vi "Start Up Procedure.vi"() -> ()   [LabVIEW 2015]
uses:
  <vilib>/DAQmx/write.llb/DAQmx Write (Digital Bool 1Line 1Point).vi
  <vilib>/DAQmx/miscellaneous.llb/DAQmx Fill In Error Info.vi
panel:
  out "PSU End of Charge":bool
  out "Start Button Pressed?":bool
  out "Earthed":bool
  out "System Reset pressed?":bool
  out "Safety System Interlock":bool
  out "HV On Relay":bool
  in  "Unlock Encloure Door":bool
  out "Enclosure Door Shut?":bool
  out "HV Enclosure OK":bool
  in  "Test HV Enclosure":bool
  out "Red Rack Enclosure OK":bool
  in  "Test Red Rack Enclosure":bool
  out "Emergency Stop OK":bool
  in  "Test Emergency Stop":bool
  out "Dump Switch Readback OK":bool
  in  "Test Dump Switch":bool
  in  "stop":bool
  out "LEDs OK":bool
  in  "Test LEDs":bool
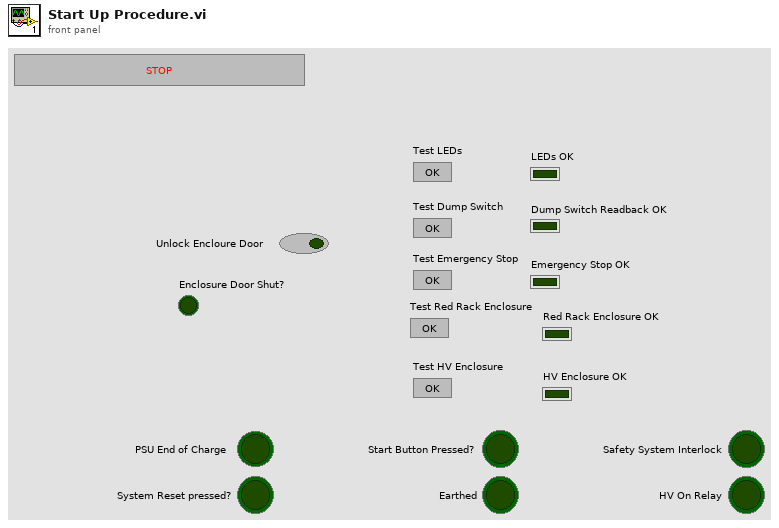
[diagram p1: front panel]
types:
  T1 = typedef "Semaphore RefNum" = refnum<k1>
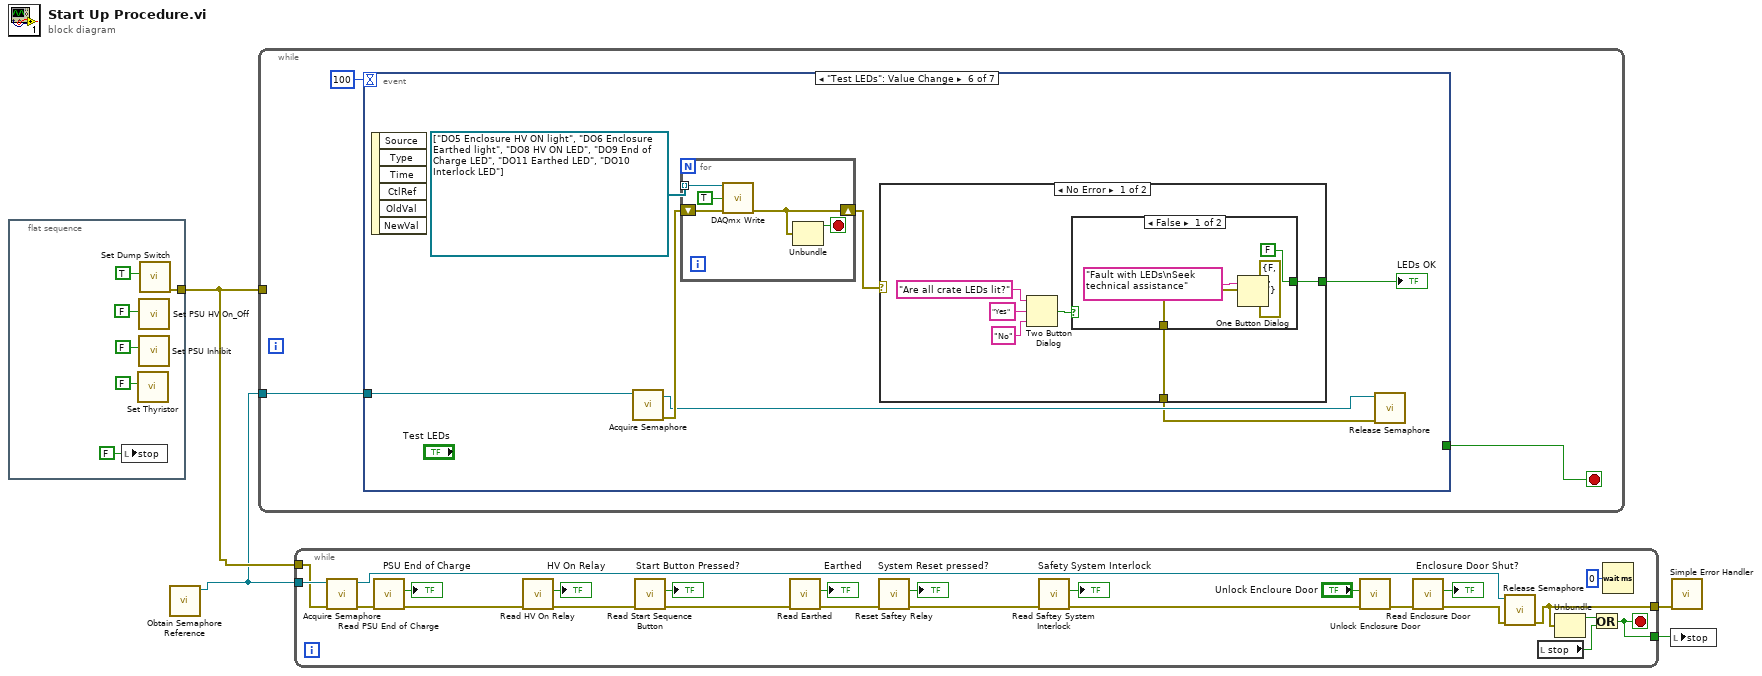
[diagram p0: block diagram]
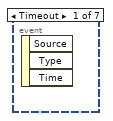
[diagram p2: hidden frame]
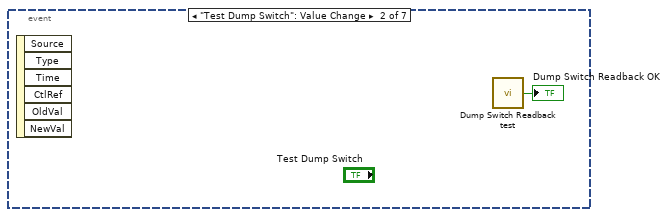
[diagram p3: hidden frame]
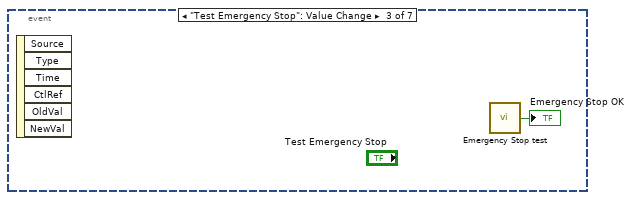
[diagram p4: hidden frame]
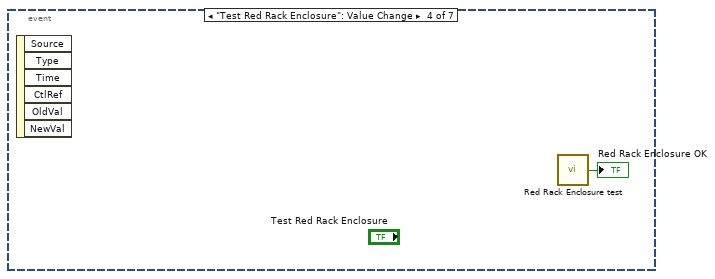
[diagram p5: hidden frame]
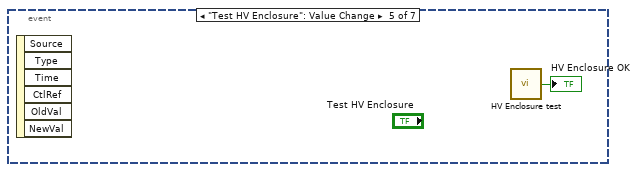
[diagram p6: hidden frame]
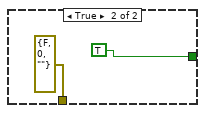
[diagram p7: hidden frame]
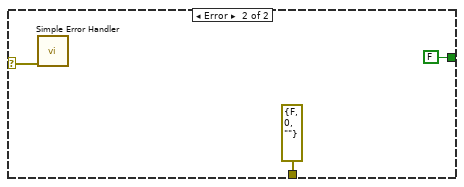
[diagram p8: hidden frame]
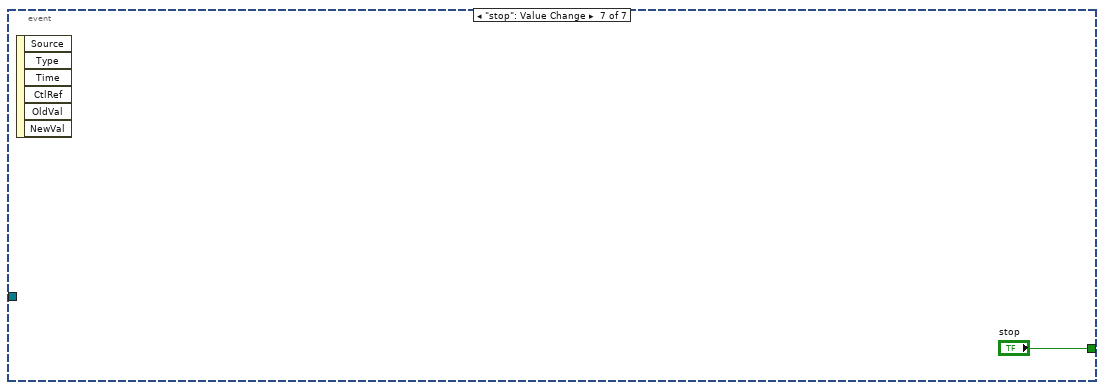
[diagram p9: hidden frame]
diagram:
  n1 = flat-sequence {
    tunnel: [w5] -> w2
    frame #0 {
      n2 = local write "stop"(FALSE ("stop")) -> ()
      n3 = call "Set Thyristor.vi"("On/Off"=FALSE ("data")) -> ()  [unwired: 6 in, 1 out]
      n4 = call "Set PSU HV On_Off.vi"("On/Off"=FALSE ("data")) -> ()  [unwired: 6 in, 1 out]
      n5 = call "Set PSU Inhibit.vi"("On/Off"=FALSE ("data")) -> ()  [unwired: 6 in, 1 out]
      n6 = call "Set Dump Switch.vi"("Earth"=TRUE) -> ("error out"=w5:errorcluster)  [unwired: 6 in]
    }
  }
  n7 = call <vilib>:"Obtain Semaphore Reference.vi"() -> ("semaphore"=w1:T1)  [unwired: 5 in, 2 out]
  n8 = while {
    tunnel: w2 -> [_]
    tunnel: w1 -> [w11]
    stop <- w12 stop-if-true
    n9 = event shown="[5] \"Test LEDs\": Value Change" {
      selector: _ -> [_ _ _ _ _ _ _]
      dyn-events: _ -> [_ _ _ _ _ _ _]
      timeout: 100 -> [_ _ _ _ _ _ _]
      tunnel: [_ _ _ _ _ _ "stop"] -> w12
      tunnel: w11 -> [_ _ _ _ _ w21 _]
      event Timeout {
        n10 = event-data() -> ()  [unwired: 1 in, 3 out]
      }
      event "Test Dump Switch": Value Change {
        n11 = event-data() -> ()  [unwired: 1 in, 6 out]
        n12 = call "Dump Switch Readback test.vi"() -> ("Dump Switch Readback OK"=→"Dump Switch Readback OK":bool)  [unwired: 2 in]
      }
      event "Test Emergency Stop": Value Change {
        n13 = event-data() -> ()  [unwired: 1 in, 6 out]
        n14 = call "Emergency Stop test.vi"() -> ("Emergency Stop OK"=→"Emergency Stop OK":bool)  [unwired: 2 in]
      }
      event "Test Red Rack Enclosure": Value Change {
        n15 = event-data() -> ()  [unwired: 1 in, 6 out]
        n16 = call "Red Rack Enclosure test.vi"() -> ("Red Rack Enclosure OK"=→"Red Rack Enclosure OK":bool)  [unwired: 2 in]
      }
      event "Test HV Enclosure": Value Change {
        n17 = event-data() -> ()  [unwired: 1 in, 6 out]
        n18 = call "HV Enclosure test.vi"() -> ("HV Enclosure OK"=→"HV Enclosure OK":bool)  [unwired: 2 in]
      }
      event "Test LEDs": Value Change {
        n19 = event-data() -> ()  [unwired: 1 in, 6 out]
        n20 = call <vilib>:"Acquire Semaphore.vi"("semaphore"=w21) -> ("error out"=w20:errorcluster, "semaphore out"=w19:T1)  [unwired: 4 in, 1 out]
        n21 = for {
          tunnel: refnum<k21>[] ["DO5 Enclosure HV ON light", "DO6 Enclosure Earthed light", "DO8 HV ON LED", "DO9 End of Charge LED", "DO11 Earthed LED", "DO10 Interlock LED"] -> [w43] mode=indexing
          shift-right: [w40] -> w23
          shift-left: w20 -> [w41]
          stop <- w39 stop-if-true
          n22 = call-poly <vilib>:"DAQmx Write.vi"("task/channels in"=w43, "data"=TRUE, "error in"=w41) -> ("error out"=w40:errorcluster)  [unwired: 10 in, 2 out]
          n23 = Unbundle(w40) -> ("status"=w39:bool)  [unwired: 2 out]
        }
        n24 = case shown="No Error" w23 {
          selector: w23 -> [_ w38]
          tunnel: [w26 FALSE ("LEDs OK")] -> w22
          tunnel: [w25 errorcluster {"status"=FALSE, "code"=0, "source"=""} ("error constant")] -> w18
          frame No Error {
            n25 = Two Button Dialog(message="Are all crate LEDs lit?", 1:"No" ("F button name (\"Cancel\")"), 2:"Yes" ("T button name (\"OK\")")) -> (T button?=w27:bool)
            n26 = case shown="False" w27 {
              tunnel: [FALSE TRUE ("LEDs OK")] -> w26
              tunnel: [errorcluster {"status"=FALSE, "code"=0, "source"=""} ("error constant") errorcluster {"status"=FALSE, "code"=0, "source"=""} ("error constant")] -> w25
              frame False {
                n27 = One Button Dialog(message="Fault with LEDs\nSeek technical assistance" ("string")) -> ()  [unwired: 1 in, 1 out]
              }
              frame True {
              }
            }
          }
          frame Error {
            n28 = call <vilib>:"Simple Error Handler.vi"("error in (no error)"=w38) -> ()  [unwired: 4 in, 5 out]
          }
        }
        "LEDs OK" <- w22
        n29 = call <vilib>:"Release Semaphore.vi"("error in (no error)"=w18, "semaphore"=w19) -> ()  [unwired: 4 in, 2 out]
      }
      event "stop": Value Change {
        n30 = event-data() -> ()  [unwired: 1 in, 6 out]
      }
    }
  }
  n31 = while {
    tunnel: [w47] -> w3
    tunnel: [w57] -> w4
    tunnel: w2 -> [w48]
    tunnel: w1 -> [w49]
    stop <- w57 stop-if-true
    n32 = call <vilib>:"Acquire Semaphore.vi"("error in (no error)"=w48, "semaphore"=w49) -> ("error out"=w50:errorcluster, "semaphore out"=w45:T1)  [unwired: 3 in, 1 out]
    n33 = call "Read PSU End of Charge.vi"("error in"=w50) -> ("error out"=w61:errorcluster, "End of Charge"=→"PSU End of Charge":bool)  [unwired: 5 in]
    n34 = call "Read HV On Relay.vi"("error in"=w61) -> ("error out"=w60:errorcluster, "HV On Relay"=→"HV On Relay":bool)  [unwired: 5 in]
    n35 = call "Read Start Sequence Button.vi"("error in"=w60) -> ("error out"=w67:errorcluster, "Start Button Pressed?"=→"Start Button Pressed?":bool)  [unwired: 5 in]
    n36 = call "Read Earthed.vi"("error in"=w67) -> ("error out"=w65:errorcluster, "Dump Switch mimic"=→"Earthed":bool)  [unwired: 5 in]
    n37 = call "Reset Saftey Relay.vi"("error in"=w65) -> ("error out"=w63:errorcluster, "System Reset pressed?"=→"System Reset pressed?":bool)  [unwired: 5 in]
    n38 = call "Read Saftey System Interlock.vi"("error in"=w63) -> ("error out"=w56:errorcluster, "Safety System Interlock"=→"Safety System Interlock":bool)  [unwired: 5 in]
    n39 = call "Unlock Enclosure Door.vi"("error in"=w56, "Unlock Encloure Door"="Unlock Encloure Door") -> ("error out"=w52:errorcluster)  [unwired: 5 in]
    n40 = call "Read Enclosure Door.vi"("error in"=w52) -> ("error out"=w46:errorcluster, "Enclosure Door Shut?"=→"Enclosure Door Shut?":bool)  [unwired: 5 in]
    n41 = call <vilib>:"Release Semaphore.vi"("error in (no error)"=w46, "semaphore"=w45) -> ("error out"=w47:errorcluster)  [unwired: 4 in, 1 out]
    n42 = local read "stop"() -> (w58:bool)
    n43 = Unbundle(w47) -> ("status"=w59:bool)  [unwired: 2 out]
    n44 = Or(x=w59, y=w58) -> (x .or. y?=w57:bool)
    n45 = Wait (ms)(milliseconds to wait=u32 0) -> ()  [unwired: 1 out]
  }
  n46 = local write "stop"(w4) -> ()
  n47 = call <vilib>:"Simple Error Handler.vi"("error in (no error)"=w3) -> ()  [unwired: 4 in, 5 out]
